vi "Teleop.vi"(10 "Match Info":T2={"Autonomous Elapsed Seconds"=0.0, "TeleOp Elapsed Seconds"=0.0, "Disabled Elapsed Seconds"=0.0, "Visited Autonomous"=FALSE, "Visited TeleOp"=FALSE, "Visited Disabled"=FALSE, "Autonomous Settings"={"Autonomous Style"=enum."Independent", "VI Refnum"=refnum}}, 11 "Call Context":T3) -> ()   [LabVIEW 2018]
doc: "This VI is called for each enabled TeleOp packet received from the DS. It is typically used to read from joysticks and other inputs and update I/O or setpoints for timed control loops. It should complete and return within 20 milliseconds or risk missing DS packets."
uses:
  <vilib>/Rock Robotics/WPI/DriverStation/WPI_DriverStationDerivedRobotMode.ctl
  <vilib>/Rock Robotics/WPI/DriverStation/WPI_DriverStationMatch Info.ctl
  <vilib>/Rock Robotics/WPI/Solenoid/WPI_SolenoidValue.ctl
  <vilib>/Rock Robotics/WPI/Utilities/WPI_GetSetVariantRefNum.vi
  <vilib>/Rock Robotics/Network Tables/NT Write Boolean Array.vi
  <vilib>/Rock Robotics/Network Tables/NT Write Numeric Array.vi
  <vilib>/Rock Robotics/Network Tables/NT Write Boolean.vi
  <vilib>/Rock Robotics/Network Tables/NT Write Number.vi
  <vilib>/Rock Robotics/WPI/RobotDrive/WPI_RobotDriveMecanumDrive_Cartesian.vi
  <vilib>/Rock Robotics/WPI/ThirdParty/Phoenix-LabVIEW/Motor Controller/Get/CTRE_Phoenix_MotorController_GetSelectedSensorData.vi
  <vilib>/Rock Robotics/WPI/Ultrasonic/WPI_SonarSRF04DigitalRefNum Registry Get.vi
  <vilib>/Rock Robotics/WPI/Ultrasonic/WPI_SonarSRF04DigitalGetRange.vi
  <vilib>/Rock Robotics/WPI/Solenoid/WPI_SolenoidSetEnum.vi
panel:
  out "YRPHfH":T1
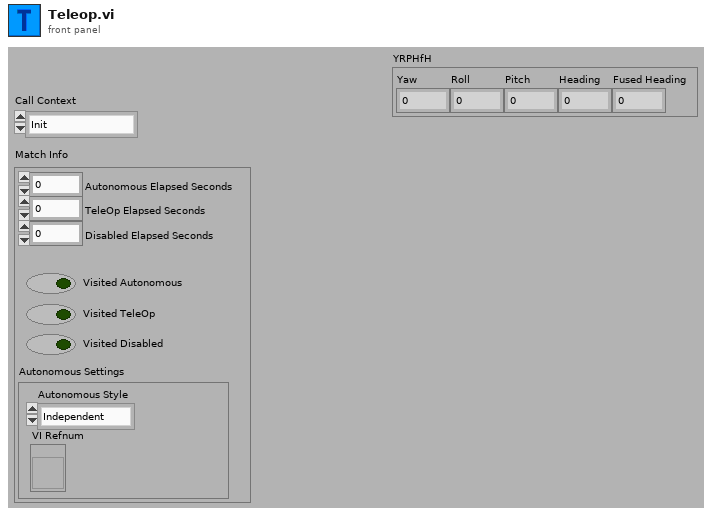
[diagram p1: front panel]
types:
  T1 = cluster{"Yaw":dbl, "Roll":dbl, "Pitch":dbl, "Heading":dbl, "Fused Heading":dbl}
  T2 = typedef "WPI_DriverStationMatch Info.ctl" = cluster{"Autonomous Elapsed Seconds":dbl, "TeleOp Elapsed Seconds":dbl, "Disabled Elapsed Seconds":dbl, "Visited Autonomous":bool, "Visited TeleOp":bool, "Visited Disabled":bool, "Autonomous Settings":cluster{"Autonomous Style":enum16{"Iterative", "Independent"}, "VI Refnum":refnum<vi>}}
  T3 = typedef "WPI_DriverStationDerivedRobotMode.ctl" = enum16{"Init", "Execute", "Stop"}
  T4 = typedef "WPI_JoystickDevRef.ctl" = cluster{"Device":T5}
  T5 = typedef "WPI_JoystickDeviceEnum.ctl" = enum16{"USB 0", "USB 1", "USB 2", "USB 3", "USB 4", "USB 5"}
  T6 = typedef "Command Status Info.ctl" = cluster{"Name":string, "Status":T7, "notifier out":T8}
  T7 = typedef "Completion Status.ctl" = enum16{"Successful", "Aborted", "Incomplete"}
  T8 = typedef "Completion Notifier.ctl" = refnum<notifier>
  T9 = typedef "WPI_MotorControlDeviceRef.ctl" = cluster{"DeviceStatus":errorcluster, "Type":T10, "PWM":cluster{"PWM Channel":T11, "DeadBand":T12}, "CAN":cluster{"Device Number":u8, "SetOutput VI Ref":variant, "GetOutput VI Ref":variant, "Enable VI Ref":variant, "Disable VI Ref":variant, "Data":variant}, "Invert":bool, "DIO PWM":cluster{"PWM \"Enable\" Channel":T11, "DIOChannel":T13, "PWM Rate":dbl}}
  T10 = typedef "WPI_MotorControlType.ctl" = enum16{"PWM", "CAN", "DIO PWM"}
  T11 = typedef "FPGA_DIOPWMChannel.ctl" = enum8{"PWM 0", "PWM 1", "PWM 2", "PWM 3", "PWM 4", "PWM 5", "PWM 6", "PWM 7", "PWM 8", "PWM 9", "PWM MXP 0", "PWM MXP 1", "PWM MXP 2", "PWM MXP 3", "PWM MXP 4", "PWM MXP 5", "PWM MXP 6", "PWM MXP 7", "PWM MXP 8", "PWM MXP 9", "Invalid"}
  T12 = typedef "WPI_PWMDeadband.ctl" = cluster{"Name":string, "maxPositivePwm":i32, "minPositivePwm":i32, "centerPwm":i32, "maxNegativePwm":i32, "minNegativePwm":i32, "angularRange":u16}
  T13 = typedef "FPGA_DIOChannel.ctl" = enum8{"DIO 0", "DIO 1", "DIO 2", "DIO 3", "DIO 4", "DIO 5", "DIO 6", "DIO 7", "DIO 8", "DIO 9", "DIO MXP 0", "DIO MXP 1", "DIO MXP 2", "DIO MXP 3", "DIO MXP 4", "DIO MXP 5", "DIO MXP 6", "DIO MXP 7", "DIO MXP 8", "DIO MXP 9", "DIO MXP 10", "DIO MXP 11", "DIO MXP 12", "DIO MXP 13", "DIO MXP 14", "DIO MXP 15", "SPI Port CS1", "SPI Port CS2", "SPI Port CS3", "SPI Port MISO", "SPI Port MOSI", "Invalid"}
  T14 = typedef "WPI_UltrasonicDeviceRef.ctl" = cluster{"DevStatus":errorcluster, "Ping Channel":T13, "Echo Channel":T13, "CntIndex":T15}
  T15 = typedef "FPGA_CounterCtrSystemIndex.ctl" = enum8{"Ctr 0", "Ctr 1", "Ctr 2", "Ctr 3", "Ctr 4", "Ctr 5", "Ctr 6", "Ctr 7", "Invalid"}
  T16 = typedef "WPI_RobotDriveDevRef.ctl" = cluster{"DevStatus":errorcluster, "Motors[]":T9[], "Square Inputs":bool, "Max Output":dbl}
  T17 = typedef "WPI_CompressorDevRef.ctl" = cluster{"DevStatus":errorcluster, "Pneumatics Control Module":u8}
  T18 = typedef "WPI_SolenoidValue.ctl" = enum16{"Off", "On", "Forward", "Reverse"}
  T19 = typedef "WPI_SolenoidDevRef.ctl" = cluster{"DevStatus":errorcluster, "Pneumatics Control Module":u8, "Forward Solenoid Channel":T20, "Reverse Solenoid Channel":T20}
  T20 = typedef "WPI_SolenoidChannel.ctl" = enum8{"Solenoid 0", "Solenoid 1", "Solenoid 2", "Solenoid 3", "Solenoid 4", "Solenoid 5", "Solenoid 6", "Solenoid 7", "Invalid"}
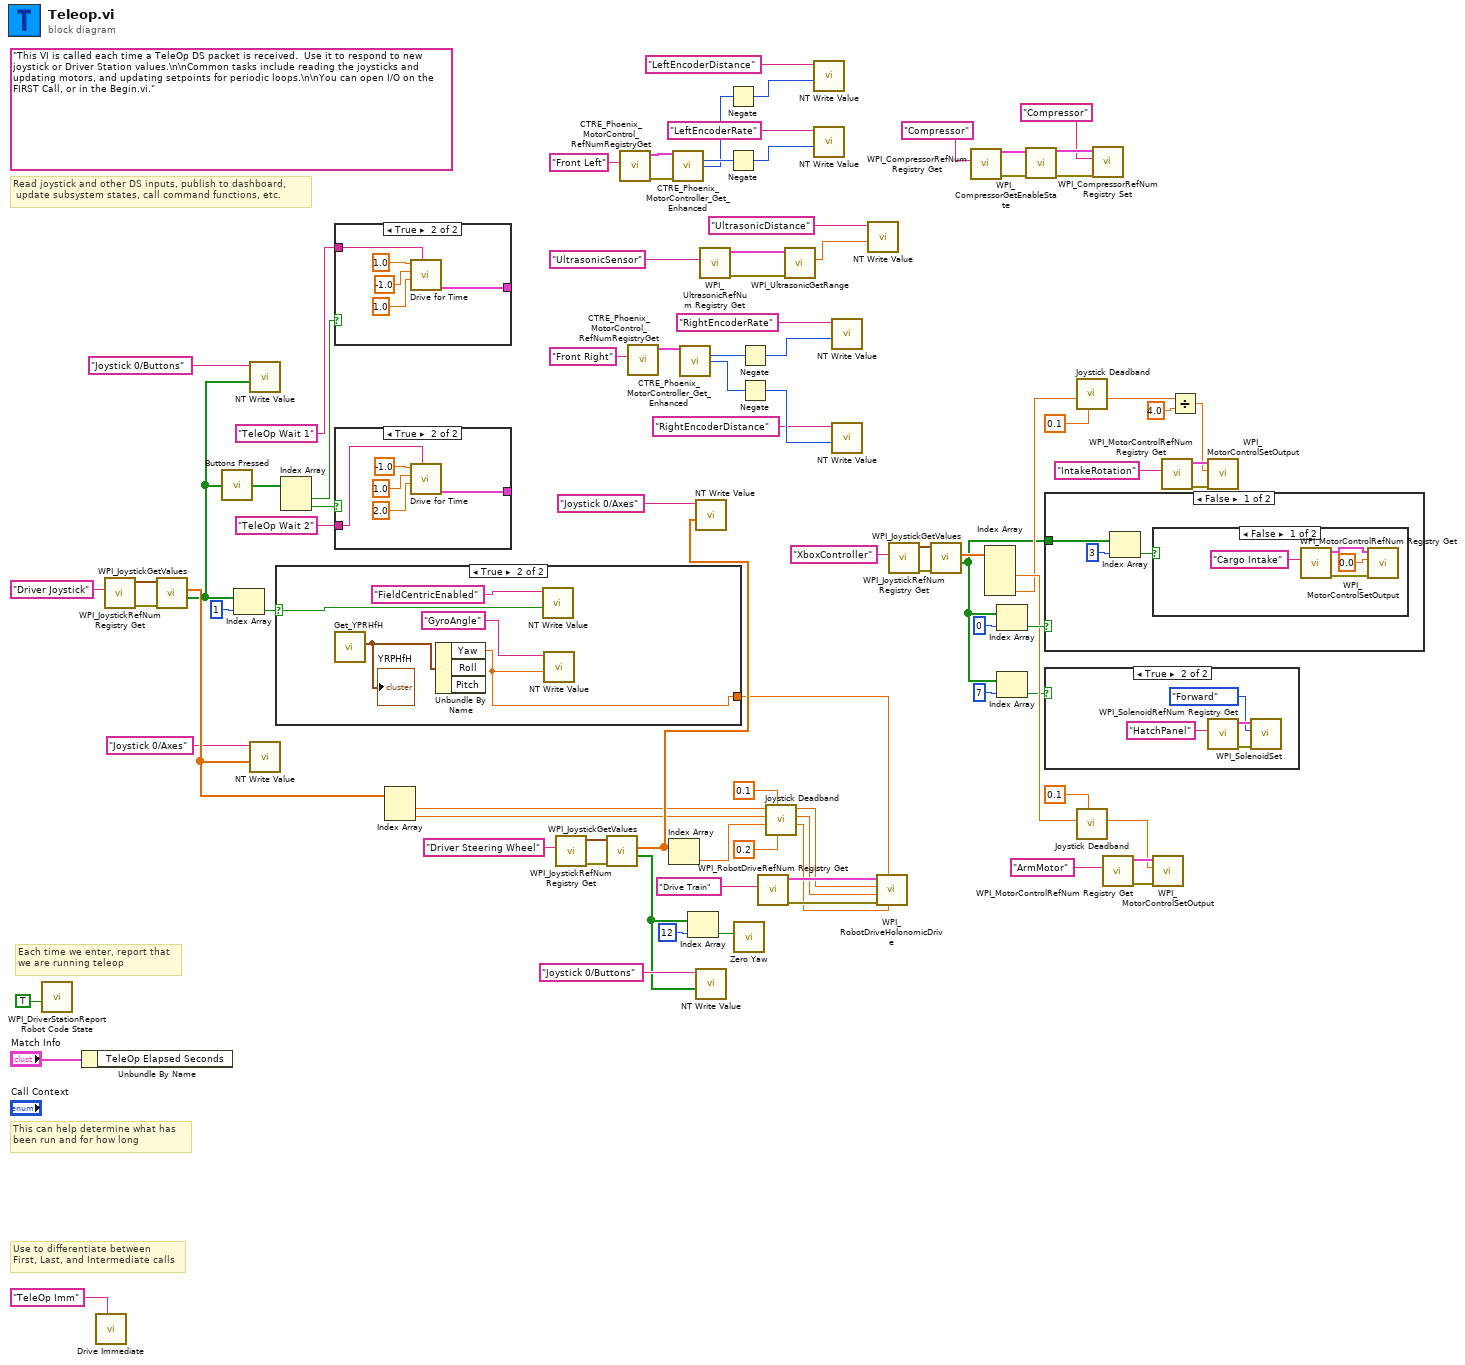
[diagram p0: block diagram]
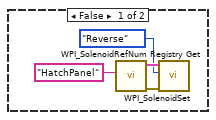
[diagram p2: hidden frame]
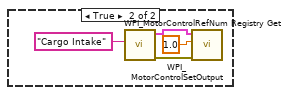
[diagram p3: hidden frame]
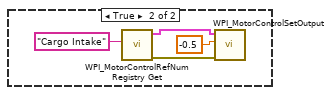
[diagram p4: hidden frame]
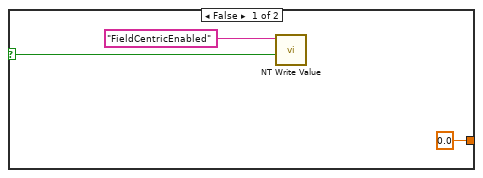
[diagram p5: hidden frame]
diagram:
  (unwired) "This VI is called each time a TeleOp DS packet is received.  Use it to respond to new joystick or Driver Station values.\n\nCommon tasks include reading the joysticks and updating motors, and updating setpoints for periodic loops.\n\nYou can open I/O on the FIRST Call, or in the Begin.vi."
  # "Read joystick and other DS inputs, publish to dashboard,\n update subsystem states, call command functions, etc."
  # "Each time we enter, report that\nwe are running teleop"
  # "Use to differentiate between\nFirst, Last, and Intermediate calls"
  # "This can help determine what has\nbeen run and for how long"
  n1 = call <vilib>:"WPI_DriverStationReport Robot Code State.vi"("TeleOp"=TRUE ("Autonomous")) -> ()  [unwired: 10 in, 1 out]
  n2 = Unbundle By Name("Match Info") -> ()  [unwired: 1 out]
  n3 = call "Drive Immediate.vi"("Description"="TeleOp Imm") -> ()  [unwired: 10 in, 1 out]
  n4 = call <vilib>:"WPI_JoystickRefNum Registry Get.vi"("refnum name"="Driver Joystick") -> ("error out"=w73:errorcluster, "JoystickDevRef"=w86:T4)  [unwired: 1 in, 8 out]
  n5 = call <vilib>:"WPI_JoystickGetValues.vi"("error in (no error)"=w73, "JoystickDevRef"=w86) -> ("Buttons"=w29:bool[], "Axes"=w78:dbl[])  [unwired: 5 in, 3 out]
  n6 = call "Buttons Pressed.vi"("Button Values"=w29) -> ("Button Presses"=w82:bool[])
  n7 = Index Array(array=w29, index=1) -> (element=w53:bool)
  n8 = call-poly <vilib>:"NT Write Value.vi"("Boolean Array"=w29, "Name"="Joystick 0/Buttons") -> ()  [unwired: 9 in, 1 out]
  n9 = call-poly <vilib>:"NT Write Value.vi"("Numeric Array"=w78, "Name"="Joystick 0/Axes") -> ()  [unwired: 9 in, 1 out]
  n10 = case shown="True" w53 {
    selector: w53 -> [w90 w96]
    tunnel: [0.0 w93] -> w54
    frame False {
      n11 = call-poly <vilib>:"NT Write Value.vi"("Boolean"=w90, "Name"="FieldCentricEnabled") -> ()  [unwired: 9 in, 1 out]
    }
    frame True {
      n12 = call <vilib>:"Get_YPRHfH.vi"() -> ("YRPHfH"=w97:T1)  [unwired: 11 in]
      "YRPHfH" <- w97
      n13 = Unbundle By Name(w97) -> ("Yaw"=w93:dbl)  [unwired: 2 out]
      n14 = call-poly <vilib>:"NT Write Value.vi"("Boolean"=w96, "Name"="FieldCentricEnabled") -> ()  [unwired: 9 in, 1 out]
      n15 = call-poly <vilib>:"NT Write Value.vi"("Numeric"=w93, "Name"="GyroAngle") -> ()  [unwired: 9 in, 1 out]
    }
  }
  n16 = Index Array(array=w82) -> (element #1=w81:bool, element #2=w80:bool)  [unwired: 2 in]
  n17 = case shown="True" w81 {
    tunnel: [_ w101] -> _
    tunnel: "TeleOp Wait 1" ("Description") -> [_ w100]
    frame False {
    }
    frame True {
      n18 = call "Drive for Time.vi"("Description"=w100, "Seconds"=1.0, "Right Speed"=-1.0, "Left Speed"=1.0) -> ("Command Info Out"=w101:T6)  [unwired: 6 in, 1 out]
    }
  }
  n19 = case shown="True" w80 {
    tunnel: [_ w105] -> _
    tunnel: "TeleOp Wait 2" ("Description") -> [_ w104]
    frame False {
    }
    frame True {
      n20 = call "Drive for Time.vi"("Description"=w104, "Seconds"=2.0, "Right Speed"=1.0, "Left Speed"=-1.0) -> ("Command Info Out"=w105:T6)  [unwired: 6 in, 1 out]
    }
  }
  n21 = Index Array(array=w78) -> (element #1=w66:dbl, element #2=w64:dbl)  [unwired: 2 in]
  n22 = call <vilib>:"WPI_JoystickRefNum Registry Get.vi"("refnum name"="Driver Steering Wheel") -> ("error out"=w75:errorcluster, "JoystickDevRef"=w74:T4)  [unwired: 9 in]
  n23 = call <vilib>:"WPI_JoystickGetValues.vi"("error in (no error)"=w75, "JoystickDevRef"=w74) -> ("Buttons"=w57:bool[], "Axes"=w70:dbl[])  [unwired: 5 in, 3 out]
  n24 = call <vilib>:"CTRE_Phoenix_MotorControl_RefNumRegistryGet.vi"("refnum name"="Front Left") -> ("error out"=w48:errorcluster, "PhoenixMotorControlDevRef"=w49:T9)  [unwired: 9 in]
  n25 = call <vilib>:"CTRE_Phoenix_MotorControl_RefNumRegistryGet.vi"("refnum name"="Front Right") -> ("PhoenixMotorControlDevRef"=w45:T9)  [unwired: 9 in, 1 out]
  n26 = Index Array(array=w70) -> (element=w62:dbl)  [unwired: 1 in]
  n27 = call-poly <vilib>:"CTRE_Phoenix_MotorController_Get_Enhanced.vi"("PhoenixMotorControlDevRef"=w49, "error in"=w48) -> ("Position (Raw Sensor Units)"=w47:i32, "Velocity (Raw Sensor Units per 100 ms)"=w37:i32)  [unwired: 10 in, 2 out]
  n28 = call-poly <vilib>:"CTRE_Phoenix_MotorController_Get_Enhanced.vi"("PhoenixMotorControlDevRef"=w45) -> ("Position (Raw Sensor Units)"=w41:i32, "Velocity (Raw Sensor Units per 100 ms)"=w40:i32)  [unwired: 11 in, 2 out]
  n29 = Index Array(array=w57, index=12) -> (element=w56:bool)
  n30 = call-poly <vilib>:"NT Write Value.vi"("Numeric Array"=w70, "Name"="Joystick 0/Axes") -> ()  [unwired: 9 in, 1 out]
  n31 = call-poly <vilib>:"NT Write Value.vi"("Boolean Array"=w57, "Name"="Joystick 0/Buttons") -> ()  [unwired: 9 in, 1 out]
  n32 = call-poly <vilib>:"WPI_UltrasonicRefNum Registry Get.vi"("refnum name"="UltrasonicSensor") -> ("error out"=w33:errorcluster, "SonarSRF04DevRef"=w34:T14)  [unwired: 9 in]
  n33 = Negate(x=w37) -> (-x=w38:i32)
  n34 = Negate(x=w47) -> (-x=w46:i32)
  n35 = call <vilib>:"Zero Yaw.vi"("Zero"=w56) -> ()  [unwired: 11 in]
  n36 = Negate(x=w41) -> (-x=w43:i32)
  n37 = Negate(x=w40) -> (-x=w42:i32)
  n38 = call <vilib>:"WPI_RobotDriveRefNum Registry Get.vi"("refnum name"="Drive Train") -> ("error out"=w69:errorcluster, "RobotDriveDevRef"=w68:T16)  [unwired: 9 in]
  n39 = call "Joystick Deadband.vi"("Z Deadband"=0.2, "X Y Deadband"=0.1, "Z"=w62, "Y"=w64, "X"=w66) -> ("Z Out"=w61:dbl, "Y Out"=w63:dbl, "X Out"=w65:dbl)  [unwired: 4 in]
  n40 = call-poly <vilib>:"WPI_UltrasonicGetRange.vi"("error in (no error)"=w33, "SonarSRF04DevRef"=w34) -> ("Distance"=w32:dbl)  [unwired: 7 in, 2 out]
  n41 = call-poly <vilib>:"NT Write Value.vi"("Numeric"=w38, "Name"="LeftEncoderDistance") -> ()  [unwired: 9 in, 1 out]
  n42 = call-poly <vilib>:"NT Write Value.vi"("Numeric"=w46, "Name"="LeftEncoderRate") -> ()  [unwired: 9 in, 1 out]
  n43 = call-poly <vilib>:"NT Write Value.vi"("Numeric"=w43, "Name"="RightEncoderRate") -> ()  [unwired: 9 in, 1 out]
  n44 = call-poly <vilib>:"NT Write Value.vi"("Numeric"=w42, "Name"="RightEncoderDistance") -> ()  [unwired: 9 in, 1 out]
  n45 = call-poly <vilib>:"NT Write Value.vi"("Numeric"=w32, "Name"="UltrasonicDistance") -> ()  [unwired: 9 in, 1 out]
  n46 = call-poly <vilib>:"WPI_RobotDriveHolonomicDrive.vi"("Rotation"=w61, "Gyro Angle"=w54, "error in (no error)"=w69, "Y"=w63, "X"=w65, "RobotDriveDevRef"=w68) -> ()  [unwired: 3 in, 3 out]
  n47 = call <vilib>:"WPI_JoystickRefNum Registry Get.vi"("refnum name"="XboxController") -> ("error out"=w27:errorcluster, "JoystickDevRef"=w26:T4)  [unwired: 9 in]
  n48 = call <vilib>:"WPI_JoystickGetValues.vi"("error in (no error)"=w27, "JoystickDevRef"=w26) -> ("Buttons"=w9:bool[], "Axes"=w22:dbl[])  [unwired: 5 in, 3 out]
  n49 = call <vilib>:"WPI_CompressorRefNum Registry Get.vi"("refnum name"="Compressor") -> ("error out"=w4:errorcluster, "CompressorDevRef"=w5:T17)  [unwired: 9 in]
  n50 = Index Array(array=w22) -> (element #2=w20:dbl, element #4=w14:dbl)  [unwired: 4 in, 2 out]
  n51 = Index Array(array=w9, index=0) -> (element=w21:bool)
  n52 = Index Array(array=w9, index=7) -> (element=w8:bool)
  n53 = call <vilib>:"WPI_CompressorGetEnableState.vi"("error in (no error)"=w4, "CompressorDevRef"=w5) -> ("error out"=w2:errorcluster, "CompressorDevRef"=w3:T17)  [unwired: 6 in, 2 out]
  n54 = case shown="False" w21 {
    tunnel: w9 -> [w109 _]
    frame False {
      n55 = Index Array(array=w109, index=3) -> (element=w108:bool)
      n56 = case shown="False" w108 {
        frame False {
          n57 = call <vilib>:"WPI_MotorControlRefNum Registry Get.vi"("refnum name"="Cargo Intake") -> ("error out"=w114:errorcluster, "MotorControlDevRef"=w113:T9)  [unwired: 9 in]
          n58 = call <vilib>:"WPI_MotorControlSetOutput.vi"("error in (no error)"=w114, "Output"=0.0, "MotorControlDevRef"=w113) -> ()  [unwired: 6 in, 3 out]
        }
        frame True {
          n59 = call <vilib>:"WPI_MotorControlRefNum Registry Get.vi"("refnum name"="Cargo Intake") -> ("error out"=w116:errorcluster, "MotorControlDevRef"=w117:T9)  [unwired: 9 in]
          n60 = call <vilib>:"WPI_MotorControlSetOutput.vi"("error in (no error)"=w116, "Output"=1.0, "MotorControlDevRef"=w117) -> ()  [unwired: 6 in, 3 out]
        }
      }
    }
    frame True {
      n61 = call <vilib>:"WPI_MotorControlRefNum Registry Get.vi"("refnum name"="Cargo Intake") -> ("error out"=w119:errorcluster, "MotorControlDevRef"=w120:T9)  [unwired: 9 in]
      n62 = call <vilib>:"WPI_MotorControlSetOutput.vi"("error in (no error)"=w119, "Output"=-0.5, "MotorControlDevRef"=w120) -> ()  [unwired: 6 in, 3 out]
    }
  }
  n63 = case shown="True" w8 {
    frame False {
      n64 = call <vilib>:"WPI_SolenoidRefNum Registry Get.vi"("refnum name"="HatchPanel") -> ("error out"=w126:errorcluster, "SolenoidDevRef"=w125:T19)  [unwired: 9 in]
      n65 = call-poly <vilib>:"WPI_SolenoidSet.vi"("error in (no error)"=w126, "Value"=WPI_SolenoidValue."Reverse", "SolenoidDevRef"=w125) -> ()  [unwired: 7 in, 2 out]
    }
    frame True {
      n66 = call <vilib>:"WPI_SolenoidRefNum Registry Get.vi"("refnum name"="HatchPanel") -> ("error out"=w130:errorcluster, "SolenoidDevRef"=w129:T19)  [unwired: 9 in]
      n67 = call-poly <vilib>:"WPI_SolenoidSet.vi"("error in (no error)"=w130, "Value"=WPI_SolenoidValue."Forward", "SolenoidDevRef"=w129) -> ()  [unwired: 7 in, 2 out]
    }
  }
  n68 = call "Joystick Deadband.vi"("Z Deadband"=0.1, "Z"=w14) -> ("Z Out"=w11:dbl)  [unwired: 7 in, 2 out]
  n69 = call "Joystick Deadband.vi"("X Y Deadband"=0.1, "Y"=w20) -> ("Y Out"=w18:dbl)  [unwired: 7 in, 2 out]
  n70 = call <vilib>:"WPI_CompressorRefNum Registry Set.vi"("error in (no error)"=w2, "refnum name"="Compressor", "CompressorDevRef"=w3) -> ()  [unwired: 7 in, 2 out]
  n71 = call <vilib>:"WPI_MotorControlRefNum Registry Get.vi"("refnum name"="ArmMotor") -> ("error out"=w24:errorcluster, "MotorControlDevRef"=w23:T9)  [unwired: 9 in]
  n72 = call <vilib>:"WPI_MotorControlSetOutput.vi"("error in (no error)"=w24, "Output"=w18, "MotorControlDevRef"=w23) -> ()  [unwired: 6 in, 3 out]
  n73 = call <vilib>:"WPI_MotorControlRefNum Registry Get.vi"("refnum name"="IntakeRotation") -> ("error out"=w17:errorcluster, "MotorControlDevRef"=w16:T9)  [unwired: 9 in]
  n74 = Divide(x=w11, y=4.0) -> (x/y=w10:dbl)
  n75 = call <vilib>:"WPI_MotorControlSetOutput.vi"("error in (no error)"=w17, "Output"=w10, "MotorControlDevRef"=w16) -> ()  [unwired: 6 in, 3 out]
